vi "_set_mixer_params.vi"(9 "_LO_P_OPT":T2={"範囲配列"=[{"Start"=1.0, "Stop"=3.5, "Step"=0.1, "ｂｙ"="NEL VG"}, {"Start"=30.0, "Stop"=75.0, "Step"=1.0, "ｂｙ"="Motor"}, {"Start"=0.5, "Stop"=2.5, "Step"=0.1, "ｂｙ"="WCA VD"}], "Optimize"=0, "file_name"="LP_914.0_Tmin_100519.csv", "Save?"=FALSE, "measure"=2, "current(uA)"=40.0, "wait(ms)"=0, "IFfrq(GHz)"=8.0, "aveg"=10, "SISparam option"=2} {"SISparam option" items=["Volt and Current", "Volt only"]; "measure" items=["Pmax (only HOT)", "Tmin (HOT/COLD)", "C current"]; "Optimize" items=["Sweep", "黄金分割"]; "範囲配列"."Step" format="%.2f"; "範囲配列"."Stop" format="%.2f"; "範囲配列"."Start" format="%.2f"}, 10 "Control":T4={"GPIB_ATT"="28", "6501Dev#"=1, "GPIB_SP"="18", "GPIB_PM"="13", "GPIB_DSA"="11", "GPIB_DMM (TPD)"="23", "GPIB_MPI"="COM12", "mortor設定"=[{"Axis"=0, "ID"=0, "HIspeed"=200.0, "LOspeed"=100.0, "ACCEL(ms)"=100.0, "Sratio"=50.0, "フリーラン\n"=FALSE, "文字列"="DSB HOT/COLD"}, {"Axis"=1, "ID"=0, "HIspeed"=4.0, "LOspeed"=4.0, "ACCEL(ms)"=100.0, "Sratio"=50.0, "フリーラン\n"=TRUE, "文字列"="SubMM Att"}, {"Axis"=0, "ID"=0, "HIspeed"=200.0, "LOspeed"=100.0, "ACCEL(ms)"=100.0, "Sratio"=50.0, "フリーラン\n"=FALSE, "文字列"="MPI Port1"}, {"Axis"=1, "ID"=0, "HIspeed"=200.0, "LOspeed"=100.0, "ACCEL(ms)"=100.0, "Sratio"=50.0, "フリーラン\n"=FALSE, "文字列"="MPI Port2"}, {"Axis"=1, "ID"=0, "HIspeed"=200.0, "LOspeed"=100.0, "ACCEL(ms)"=100.0, "Sratio"=50.0, "フリーラン\n"=TRUE, "文字列"="gainComp"}], "DATAパス"=path "C:/Documents and Settings/band10/デスクトップ/data/cartridge/SN07/CCA07-11/120710_DSB", "mixer param file  "=path "C:/Documents and Settings/band10/デスクトップ/data/cartridge/SN07/120710_CCA07-11_mikxparam.csv", "comment"="120710_CCA07-11_DSB", "ColdCarts"="B10-07.11", "Th"=300.0, "Tc"=83.94, "Set_SIS_volt"=1.9, "Offset"=0.0, "control"=0, "FreqLO"=826.0, "Set_Mag_Cur"=9.66058394160584, "MPI offset(mm)"=23.128, "HOT/COLD"=0} {"HOT/COLD" items=["DSB", "SBR (Cart.)", "GainComp", "SBR (MIX)"]; "control" items=["CLOSE LOOP", "OPEN LOOP", "Not Control"]}, 11 "Bias_LO_equip":T3={"Node address"=19, "CAN Interface"="CAN0", "Cartridge band"=10, "Slave Node in"={"Address"=19, "Serial Number"=[16, 98, 22, 85, 1, 8, 0, 50]}, "ObjHandle out"=21, "POL"=1, "sb"=1, "GPIB_SM (SIS S,V)"="24", "GPIB_DMM (SIS I)"="22", "GPIB_SM (MAG I) "="25", "GPIB_SG(LO)"="19", "GPIB_PW (PAMP) "="6", "GPIB_TMP1(8ch)"="12", "GPIB_TMP2(2ch)  "="13", "WCA_avg"=10, "Rsen"=10.0, "BiasModule"=1, "LOModule "=2, "WCA_LO_FREQ_SET"={"YTO Low freq. [GHz]"=14.65, "YTO High freq. [GHz]"=17.5, "Kvco"=1, "Lock Pol."=0, "SET LO FREQ"=91.77778, "Multiplier"=6.0, "YTO (HEX)"=934, "YTO ( FREQ)"=15.300036, "NULL PLL INTEGRATOR"=FALSE}, "Res for"=0} {"Res for" items=["none", "series res", "parallel res"]; "WCA_LO_FREQ_SET"."YTO ( FREQ)" min=25 max=150 step=0.0001 format="%.3f"; "WCA_LO_FREQ_SET"."Multiplier" min=3 max=6 step=3; "WCA_LO_FREQ_SET"."SET LO FREQ" min=25 max=150 step=0.0001 format="%.3f"; "WCA_LO_FREQ_SET"."Lock Pol." items=["Lower", "Upper"]; "WCA_LO_FREQ_SET"."Kvco" items=["7.5MHz/V", "15MHz/V"]; "WCA_LO_FREQ_SET"."YTO High freq. [GHz]" format="%.3f"; "WCA_LO_FREQ_SET"."YTO Low freq. [GHz]" format="%.3f"; "LOModule" items=["Manual Gunn+PAMP"=0, "PLL GUNN+PAMP"=5, "B10Lab LO"=1, "WCA LO"=2, ""=3, "YIG発信器"=4, "none"=99]; "BiasModule" items=["B10Lab Bias"=0, "WCA BiasModule"=1, "none"=99]; "Slave Node in"."Serial Number" format="%.0x"; "Slave Node in"."Address" format="%.0x"; "Cartridge band" max=10 step=1; "Node address" format="%.0x"}) -> (1 "文字列":string="LOPt,826.00,1.31,1.84,21.22,-18.26,-21.13,146.13,19.78,,WCA,1.825867,205.642700,-0.241241,  3.501740,349.212646,-0.243988,", 2 "Control 2":T1={"GPIB_ATT"="28", "6501Dev#"=1, "GPIB_SP"="18", "GPIB_PM"="13", "GPIB_DSA"="11", "GPIB_DMM (TPD)"="23", "GPIB_MPI"="COM12", "mortor設定"=[{"Axis"=0, "ID"=0, "HIspeed"=200.0, "LOspeed"=100.0, "ACCEL(ms)"=100.0, "Sratio"=50.0, "フリーラン\n"=FALSE, "文字列"="DSB HOT/COLD"}, {"Axis"=1, "ID"=0, "HIspeed"=4.0, "LOspeed"=4.0, "ACCEL(ms)"=100.0, "Sratio"=50.0, "フリーラン\n"=TRUE, "文字列"="SubMM Att"}, {"Axis"=0, "ID"=0, "HIspeed"=200.0, "LOspeed"=100.0, "ACCEL(ms)"=100.0, "Sratio"=50.0, "フリーラン\n"=FALSE, "文字列"="MPI Port1"}, {"Axis"=1, "ID"=0, "HIspeed"=200.0, "LOspeed"=100.0, "ACCEL(ms)"=100.0, "Sratio"=50.0, "フリーラン\n"=FALSE, "文字列"="MPI Port2"}, {"Axis"=1, "ID"=0, "HIspeed"=200.0, "LOspeed"=100.0, "ACCEL(ms)"=100.0, "Sratio"=50.0, "フリーラン\n"=TRUE, "文字列"="gainComp"}], "DATAパス"=path "C:/Documents and Settings/band10/デスクトップ/data/cartridge/SN07/CCA07-11/120710_DSB", "DBパス "=path "C:/Documents and Settings/band10/デスクトップ/data/cartridge/SN07/120710_CCA07-11_mikxparam.csv", "comment"="120710_CCA07-11_DSB", "ColdCarts"="B10-07.11", "Th"=300.0, "Tc"=83.94, "Set_SIS_volt"=1.9, "Offset"=0.0, "control"=0, "FreqLO"=826.0, "Set_Mag_Cur"=9.66058394160584, "MPI offset(mm)"=23.128, "HOT/COLD"=0} {"HOT/COLD" items=["DSB", "SBR (Cart.)", "GainComp", "SBR (MIX)"]; "control" items=["CLOSE LOOP", "OPEN LOOP", "Not Control"]}, 3 "Bias_LO_equip 2":T3={"Node address"=19, "CAN Interface"="CAN0", "Cartridge band"=10, "Slave Node in"={"Address"=19, "Serial Number"=[16, 98, 22, 85, 1, 8, 0, 50]}, "ObjHandle out"=21, "POL"=1, "sb"=1, "GPIB_SM (SIS S,V)"="24", "GPIB_DMM (SIS I)"="22", "GPIB_SM (MAG I) "="25", "GPIB_SG(LO)"="19", "GPIB_PW (PAMP) "="6", "GPIB_TMP1(8ch)"="12", "GPIB_TMP2(2ch)  "="13", "WCA_avg"=10, "Rsen"=10.0, "BiasModule"=1, "LOModule "=2, "WCA_LO_FREQ_SET"={"YTO Low freq. [GHz]"=14.65, "YTO High freq. [GHz]"=17.5, "Kvco"=1, "Lock Pol."=0, "SET LO FREQ"=91.77778, "Multiplier"=6.0, "YTO (HEX)"=934, "YTO ( FREQ)"=15.300036, "NULL PLL INTEGRATOR"=FALSE}, "Res for"=0} {"Res for" items=["none", "series res", "parallel res"]; "WCA_LO_FREQ_SET"."YTO ( FREQ)" min=25 max=150 step=0.0001 format="%.4f"; "WCA_LO_FREQ_SET"."Multiplier" min=3 max=6 step=3; "WCA_LO_FREQ_SET"."SET LO FREQ" min=25 max=150 step=0.0001 format="%.3f"; "WCA_LO_FREQ_SET"."Lock Pol." items=["Lower", "Upper"]; "WCA_LO_FREQ_SET"."Kvco" items=["7.5MHz/V", "15MHz/V"]; "WCA_LO_FREQ_SET"."YTO High freq. [GHz]" format="%.3f"; "WCA_LO_FREQ_SET"."YTO Low freq. [GHz]" format="%.3f"; "LOModule" items=["Manual", "B10Lab LO", "WCA LO"]; "BiasModule" items=["B10Lab Bias", "WCA BiasModule"]; "Slave Node in"."Serial Number" format="%.0x"; "Slave Node in"."Address" format="%.0x"; "Cartridge band" max=10 step=1; "Node address" format="%.0x"})   [LabVIEW 2017]
uses:
  WCA_NAOJ_sub_vi/WCA_Global.vi
  <vilib>/Utility/file.llb/Read From Spreadsheet File (string).vi
  <vilib>/gmath/NI_Gmath.lvlib
panel:
  out "配列":string[][](array[string])=[["MixerParam", "4.46", "794", " 2012-07-10  09:04:23", "1.79", "41", "9.9", "", "", "1", "2", "1", "1.85", "0", "10.2", "0.32"], ["MixerParam", "4.46", "799", " 2012-07-10  09:09:38", "1.79", "41", "9.9", "", "", "1", "2", "1", "1.85", "0", "10.2", "0.32"], ["MixerParam", "4.46", "802", " 2012-07-10  09:14:53", "1.79", "41", "9.9", "", "", "1", "2", "1", "1.85", "0", "10.2", "0.32"], ["MixerParam", "4.46", "810", " 2012-07-10  09:20:08", "1.84", "41", "9.9", "", "", "1", "2", "1", "1.9", "0", "10.2", "0.32"], ["MixerParam", "4.46", "818", " 2012-07-10  09:25:23", "1.84", "41", "9.9", "", "", "1", "2", "1", "1.9", "0", "10.2", "0.32"], ["MixerParam", "4.46", "826", " 2012-07-10  09:30:38", "1.84", "41", "9.9", "", "", "1", "2", "1", "1.9", "0", "10.2", "0.33"], ["MixerParam", "4.46", "834", " 2012-07-10  09:35:53", "1.89", "41", "9.9", "", "", "1", "2", "1", "1.95", "0", "10.2", "0.32"], ["MixerParam", "4.46", "842", " 2012-07-10  09:41:08", "1.89", "41", "9.9", "", "", "1", "2", "1", "1.95", "0", "10.2", "0.33"], ["MixerParam", "4.47", "850", " 2012-07-10  09:46:24", "1.89", "41", "9.9", "", "", "1", "2", "1", "1.95", "0", "10.2", "0.32"], ["MixerParam", "4.46", "858", " 2012-07-10  09:51:42", "1.89", "41", "9.9", "", "", "1", "2", "1", "1.95", "0", "10.2", "0.32"], ["MixerParam", "4.46", "866", " 2012-07-10  09:56:58", "1.94", "41", "9.9", "", "", "1", "2", "1", "2", "0", "10.2", "0.32"], ["MixerParam", "4.46", "874", " 2012-07-10  10:02:15", "1.94", "41", "9.9", "", "", "1", "2", "1", "2", "0", "10.2", "0.32"], ["MixerParam", "4.46", "882", " 2012-07-10  10:07:32", "1.94", "41", "9.9", "", "", "1", "2", "1", "2", "0", "10.2", "0.32"], ["MixerParam", "4.47", "890", " 2012-07-10  10:12:49", "1.94", "41", "9.9", "", "", "1", "2", "1", "2", "0", "10.2", "0.32"], ["MixerParam", "4.46", "893", " 2012-07-10  10:18:06", "1.98", "41", "9.9", "", "", "1", "2", "1", "2.05", "0", "10.2", "0.32"], ["MixerParam", "4.46", "898", " 2012-07-10  10:23:23", "2", "41", "9.9", "", "", "1", "2", "1", "2.05", "0", "10.2", "0.32"], ["MixerParam", "4.46", "906", " 2012-07-10  10:28:43", "2", "41", "9.9", "", "", "1", "2", "1", "2.05", "0", "10.2", "0.32"], ["MixerParam", "4.46", "914", " 2012-07-10  10:34:01", "1.99", "41", "9.9", "", "", "1", "2", "1", "2.05", "0", "10.2", "0.33"], ["MixerParam", "4.46", "922", " 2012-07-10  10:39:20", "2.04", "41", "9.9", "", "", "1", "2", "1", "2.1", "0", "10.2", "0.32"], ["MixerParam", "4.46", "930", " 2012-07-10  10:44:38", "2.04", "41", "9.9", "", "", "1", "2", "1", "2.1", "0", "10.2", "0.32"], ["MixerParam", "4.46", "938", " 2012-07-10  10:49:56", "2.04", "41", "9.9", "", "", "1", "2", "1", "2.1", "0", "10.2", "0.32"]]
  out "set I":dbl=41.0
  out "set offset":dbl
  out "setV":dbl=1.9
  out "offset":dbl[](array[numeric])
  out "I":dbl[](array[numeric])=[41.0, 41.0, 41.0, 41.0, 41.0, 41.0, 41.0, 41.0, 41.0, 41.0, 41.0, 41.0, 41.0, 41.0, 41.0, 41.0, 41.0, 41.0, 41.0, 41.0, 41.0]
  out "V":dbl[](array[numeric])=[1.85, 1.85, 1.85, 1.9, 1.9, 1.9, 1.95, 1.95, 1.95, 1.95, 2.0, 2.0, 2.0, 2.0, 2.05, 2.05, 2.05, 2.05, 2.1, 2.1, 2.1]
  out "LO":dbl[](array[numeric])=[794.0, 799.0, 802.0, 810.0, 818.0, 826.0, 834.0, 842.0, 850.0, 858.0, 866.0, 874.0, 882.0, 890.0, 893.0, 898.0, 906.0, 914.0, 922.0, 930.0, 938.0]
  out "Link済み":bool=TRUE
  # "LO freq. [GHz]"
  # "YTO LOW\n/High Freq."
  # "ZERO Intgrtr"
  # "Node Address"
  # "Serial Number"
  # "LO freq. [GHz]"
  # "YTO LOW\n/High Freq."
  # "ZERO Intgrtr"
  # "Node Address"
  # "Serial Number"
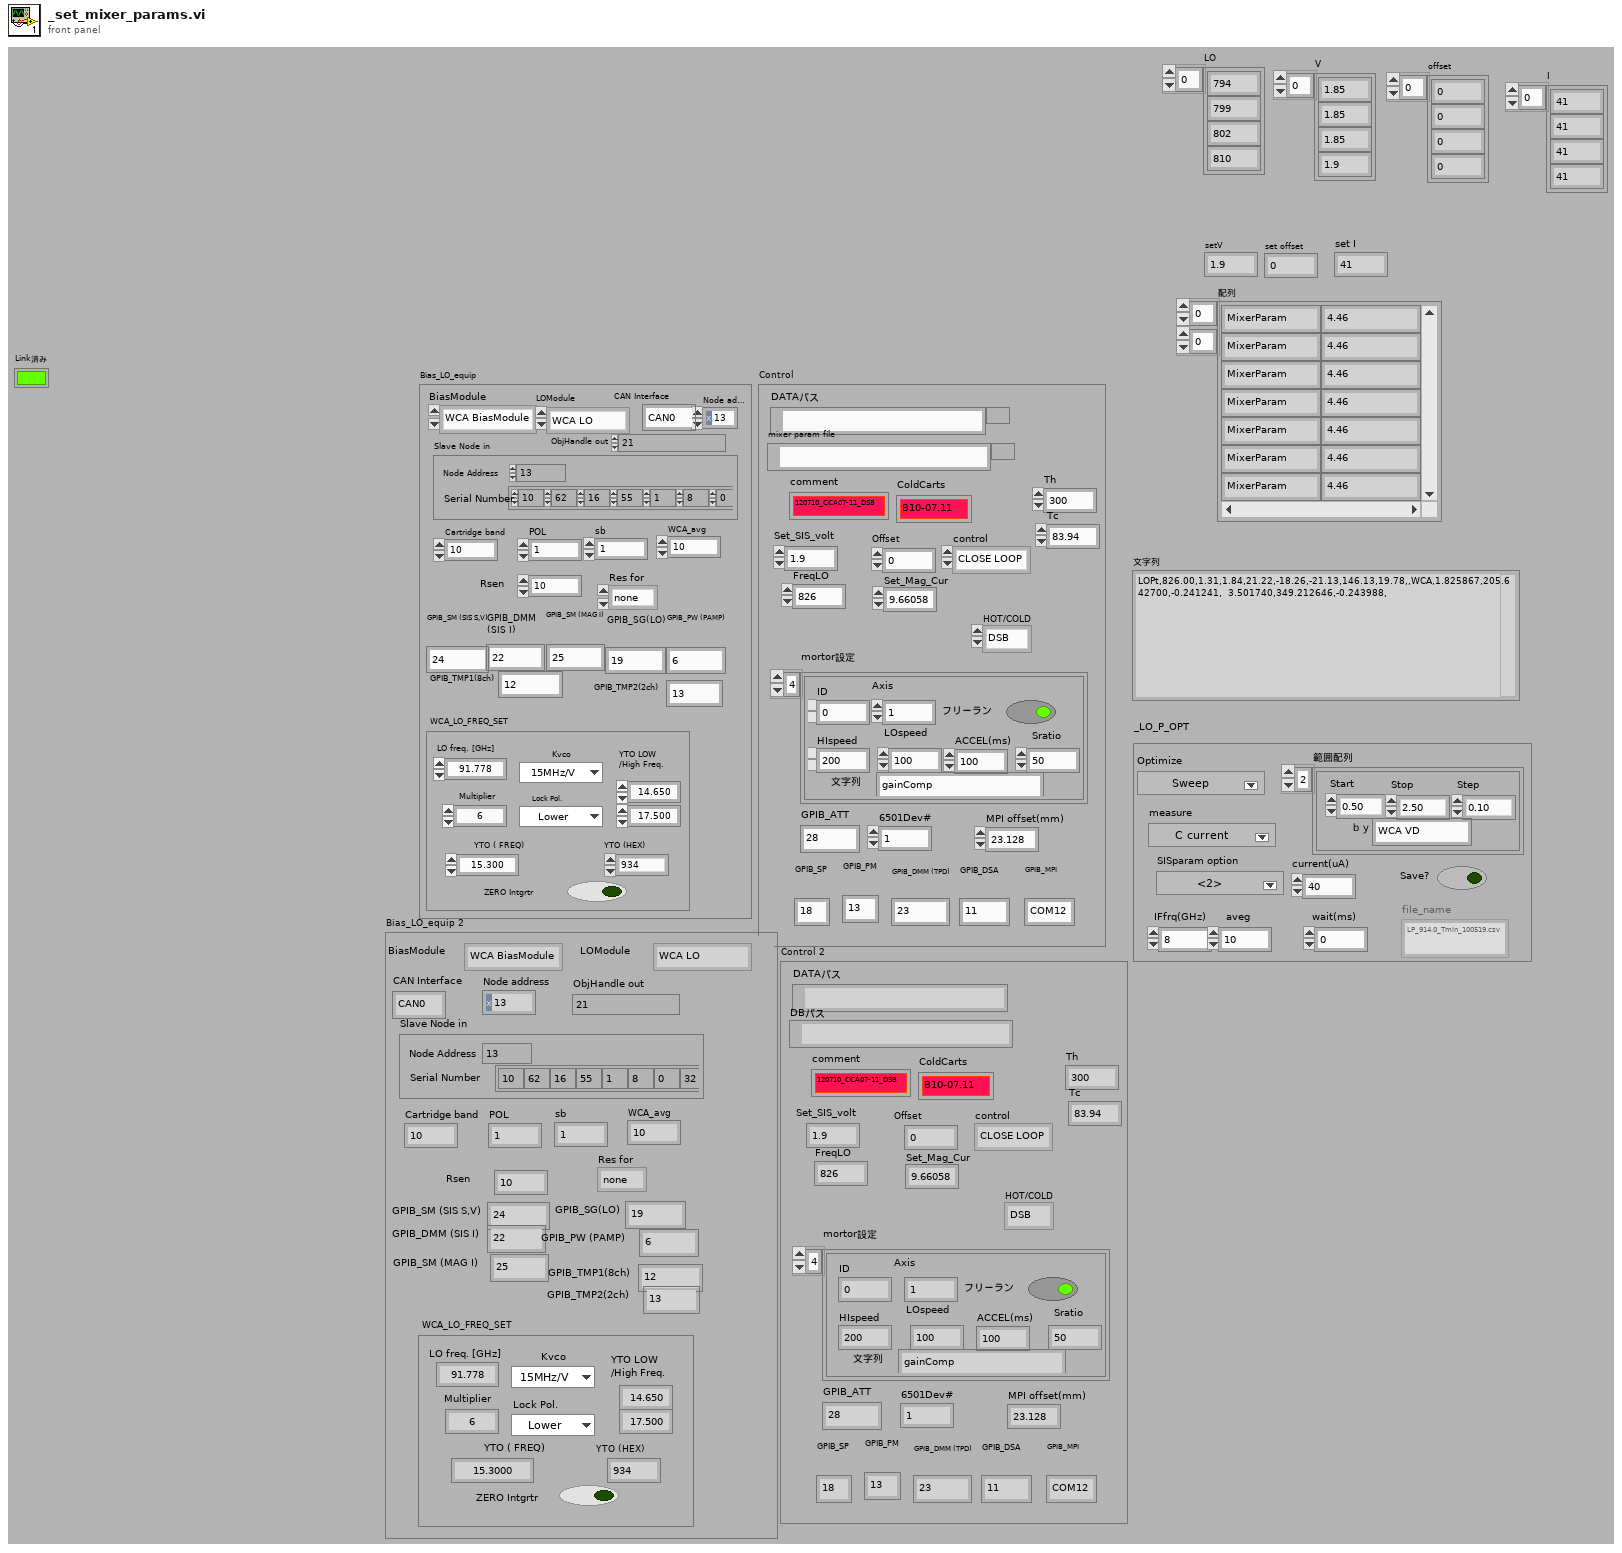
[diagram p1: front panel]
types:
  T1 = cluster{"GPIB_ATT":string, "6501Dev#":i16, "GPIB_SP":string, "GPIB_PM":string, "GPIB_DSA":string, "GPIB_DMM (TPD)":string, "GPIB_MPI":string, "mortor設定":cluster{"Axis":i16, "ID":i16, "HIspeed":dbl, "LOspeed":dbl, "ACCEL(ms)":dbl, "Sratio":dbl, "フリーラン\n":bool, "文字列":string}[], "DATAパス":path, "DBパス ":path, "comment":string, "ColdCarts":string, "Th":dbl, "Tc":dbl, "Set_SIS_volt":dbl, "Offset":dbl, "control":u16, "FreqLO":dbl, "Set_Mag_Cur":dbl, "MPI offset(mm)":dbl, "HOT/COLD":u16}
  T2 = cluster{"範囲配列":cluster{"Start":dbl, "Stop":dbl, "Step":dbl, "ｂｙ":string}[], "Optimize":u16, "file_name":string, "Save?":bool, "measure":u16, "current(uA)":dbl, "wait(ms)":i32, "IFfrq(GHz)":dbl, "aveg":i32, "SISparam option":u16}
  T3 = cluster{"Node address":u16, "CAN Interface":string, "Cartridge band":u32, "Slave Node in":cluster{"Address":i16, "Serial Number":i8[]}, "ObjHandle out":u32, "POL":u32, "sb":u32, "GPIB_SM (SIS S,V)":string, "GPIB_DMM (SIS I)":string, "GPIB_SM (MAG I) ":string, "GPIB_SG(LO)":string, "GPIB_PW (PAMP) ":string, "GPIB_TMP1(8ch)":string, "GPIB_TMP2(2ch)  ":string, "WCA_avg":i32, "Rsen":dbl, "BiasModule":u16, "LOModule ":u16, "WCA_LO_FREQ_SET":cluster{"YTO Low freq. [GHz]":sgl, "YTO High freq. [GHz]":sgl, "Kvco":u16, "Lock Pol.":u16, "SET LO FREQ":sgl, "Multiplier":sgl, "YTO (HEX)":u16, "YTO ( FREQ)":sgl, "NULL PLL INTEGRATOR":bool}, "Res for":u16}
  T4 = cluster{"GPIB_ATT":string, "6501Dev#":i16, "GPIB_SP":string, "GPIB_PM":string, "GPIB_DSA":string, "GPIB_DMM (TPD)":string, "GPIB_MPI":string, "mortor設定":cluster{"Axis":i16, "ID":i16, "HIspeed":dbl, "LOspeed":dbl, "ACCEL(ms)":dbl, "Sratio":dbl, "フリーラン\n":bool, "文字列":string}[], "DATAパス":path, "mixer param file  ":path, "comment":string, "ColdCarts":string, "Th":dbl, "Tc":dbl, "Set_SIS_volt":dbl, "Offset":dbl, "control":u16, "FreqLO":dbl, "Set_Mag_Cur":dbl, "MPI offset(mm)":dbl, "HOT/COLD":u16}
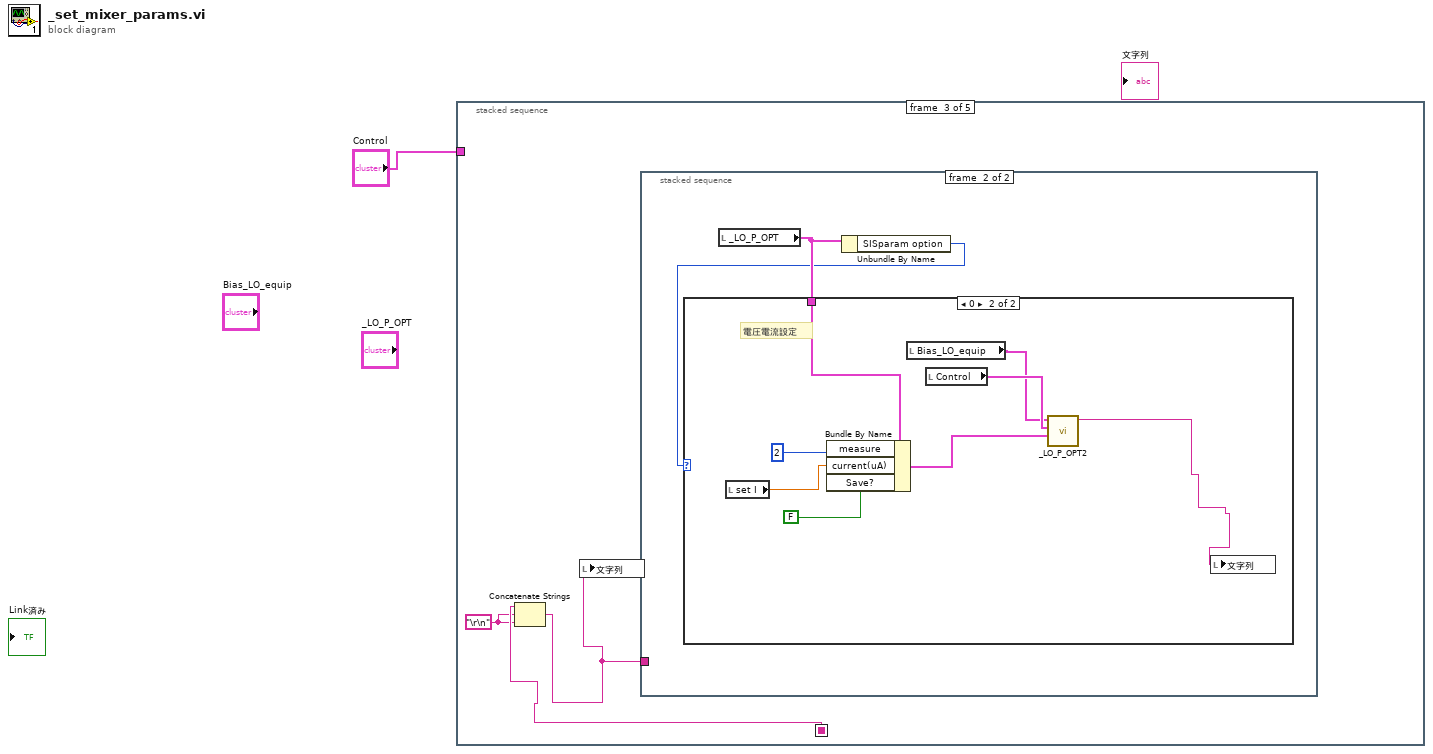
[diagram p0: block diagram]
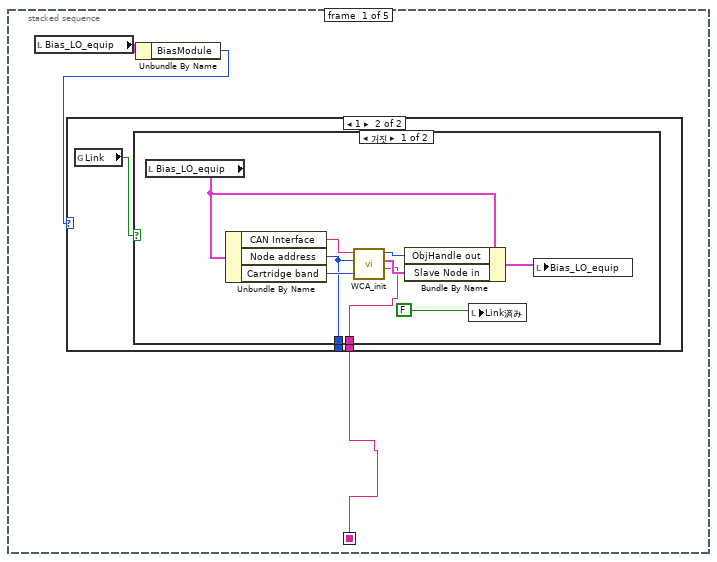
[diagram p2: hidden frame]
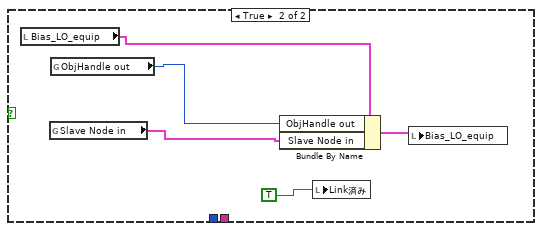
[diagram p4: hidden frame]
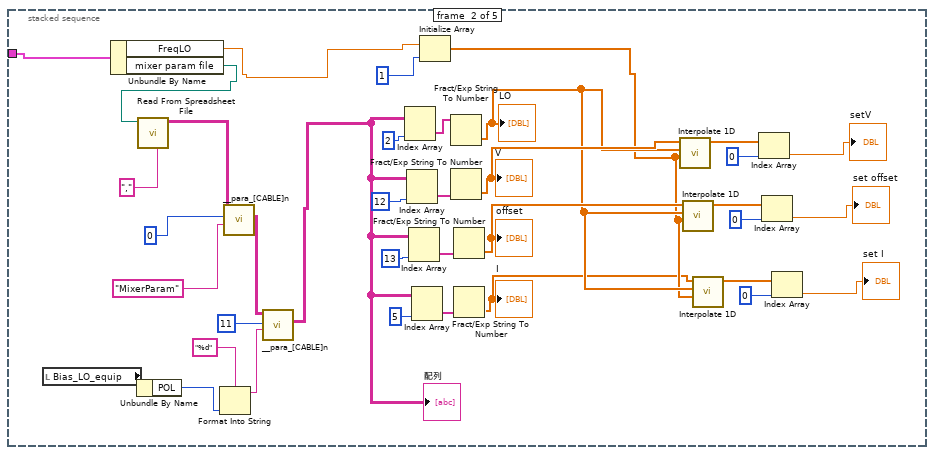
[diagram p5: hidden frame]
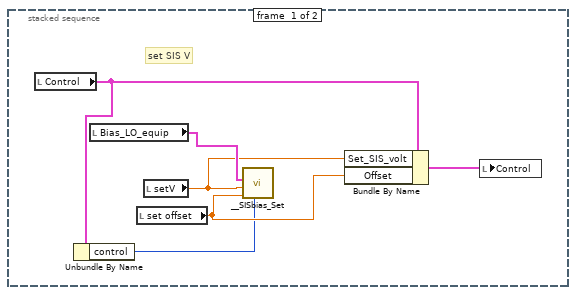
[diagram p6: hidden frame]
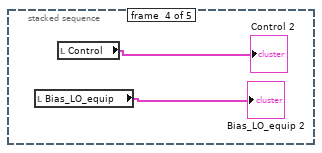
[diagram p8: hidden frame]
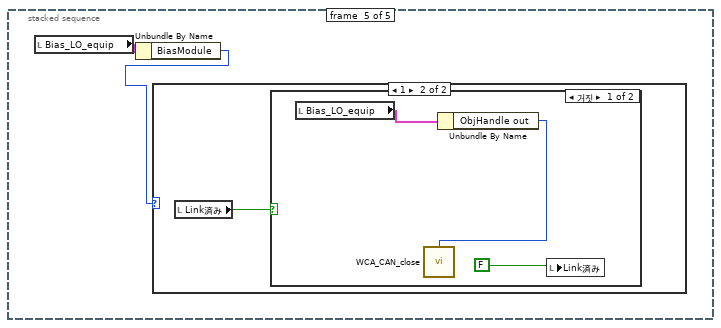
[diagram p9: hidden frame]
diagram:
  n1 = stacked-sequence {
    seq-local: [w2 _ _ _ _] -> [_ _ w61 _ _]
    tunnel: "Control" -> [_ w27 _ _ _]
    frame #0 {
      n2 = local read "Bias_LO_equip"() -> (w4:T3)
      n3 = Unbundle By Name(w4) -> ("BiasModule"=w3:u16)
      n4 = case shown="1" w3 {
        tunnel: [_ w6] -> w2
        tunnel: [_ w5] -> _
        frame 0, Default {
        }
        frame 1 {
          n5 = global read "WCA_Global.vi" "Link"() -> (w7:bool)
          n6 = case shown="거짓" w7 {
            tunnel: [w8 _] -> w6
            tunnel: [w9 _] -> w5
            frame False {
              n7 = local read "Bias_LO_equip"() -> (w10:T3)
              n8 = Unbundle By Name(w10) -> ("CAN Interface"=w13:string, "Node address"=w9:u16, "Cartridge band"=w12:u32)
              n9 = call "WCA_init.vi"("Cartridge band"=w12, "Node address"=w9, "CAN Interface"=w13) -> ("Detected CAN Nodes."=w8:string, "Slave Node in"=w15:cluster{"Address":i16, "Serial Number":i8[]}, "ObjHandle out"=w16:u32)  [unwired: 4 in, 2 out]
              n10 = Bundle By Name(cluster=w10, "ObjHandle out"=w16, "Slave Node in"=w15) -> (w11:T3)
              n11 = local write "Link済み"(FALSE) -> ()
              n12 = local write "Bias_LO_equip"(w11) -> ()
            }
            frame True {
              n13 = local read "Bias_LO_equip"() -> (w20:T3)
              n14 = global read "WCA_Global.vi" "Slave Node in"() -> (w18:cluster{"Address":i16, "Serial Number":i8[]})
              n15 = global read "WCA_Global.vi" "ObjHandle out"() -> (w19:u32)
              n16 = Bundle By Name(cluster=w20, "ObjHandle out"=w19, "Slave Node in"=w18) -> (w21:T3)
              n17 = local write "Link済み"(TRUE) -> ()
              n18 = local write "Bias_LO_equip"(w21) -> ()
            }
          }
        }
      }
    }
    frame #1 {
      n19 = local read "Bias_LO_equip"() -> (w32:T3)
      n20 = Unbundle By Name(w27) -> ("FreqLO"=w26:dbl, "mixer param file"=w22:path)
      n21 = Unbundle By Name(w32) -> ("POL"=w31:u32)
      n22 = call-poly <vilib>:"Read From Spreadsheet File.vi"("delimiter (\\t)"=",", "file path (dialog if empty)"=w22) -> ("all rows"=w37:string[][])  [unwired: 5 in, 4 out]
      n23 = Format Into String(format string="%d", w31) -> (resulting string=w29:string)  [unwired: 2 in, 1 out]
      n24 = call "__para_[CABLE]n.vi"("検索値"="MixerParam", "検索キー列"=0, "読み込み配列"=w37) -> ("出力配列"=w34:string[][])  [unwired: 6 in]
      n25 = call "__para_[CABLE]n.vi"("検索値"=w29, "検索キー列"=11, "読み込み配列"=w34) -> ("出力配列"=w33:string[][])  [unwired: 6 in]
      "配列" <- w33
      n26 = Index Array(array=w33, index (col)=2) -> (element=w56:string[])  [unwired: 1 in]
      n27 = Index Array(array=w33, index (col)=12) -> (element=w54:string[])  [unwired: 1 in]
      n28 = Index Array(array=w33, index (col)=13) -> (element=w50:string[])  [unwired: 1 in]
      n29 = Index Array(array=w33, index (col)=5) -> (element=w52:string[])  [unwired: 1 in]
      n30 = Initialize Array(w26, 1) -> (w39:dbl[])
      n31 = Fract/Exp String To Number(string=w56) -> (number=w40:dbl[])  [unwired: 3 in, 1 out]
      "LO" <- w40
      n32 = Fract/Exp String To Number(string=w54) -> (number=w49:dbl[])  [unwired: 3 in, 1 out]
      "V" <- w49
      n33 = Fract/Exp String To Number(string=w50) -> (number=w41:dbl[])  [unwired: 3 in, 1 out]
      "offset" <- w41
      n34 = Fract/Exp String To Number(string=w52) -> (number=w38:dbl[])  [unwired: 3 in, 1 out]
      "I" <- w38
      n35 = call <vilib>:"Interpolate 1D.vi"("xi"=w39, "X"=w40, "Y"=w49) -> ("yi"=w48:dbl[])  [unwired: 6 in, 2 out]
      n36 = call <vilib>:"Interpolate 1D.vi"("xi"=w39, "X"=w40, "Y"=w41) -> ("yi"=w45:dbl[])  [unwired: 6 in, 2 out]
      n37 = call <vilib>:"Interpolate 1D.vi"("xi"=w39, "X"=w40, "Y"=w38) -> ("yi"=w43:dbl[])  [unwired: 6 in, 2 out]
      n38 = Index Array(array=w48, index=0) -> (element=→"setV":dbl)
      n39 = Index Array(array=w45, index=0) -> (element=→"set offset":dbl)
      n40 = Index Array(array=w43, index=0) -> (element=→"set I":dbl)
    }
    frame #2 {
      w60 = "\r\n"
      n41 = Concatenate Strings(w61, w60, w60) -> (w59:string)
      n42 = local write "文字列"(w59) -> ()
      n43 = stacked-sequence {
        tunnel: w59 -> [_ _]
        frame #0 {
          # "set SIS V"
          n44 = local read "Control"() -> (w63:T4)
          n45 = Unbundle By Name(w63) -> ("control"=w62:u16)
          n46 = local read "Bias_LO_equip"() -> (w67:T3)
          n47 = local read "set offset"() -> (w64:dbl)
          n48 = local read "setV"() -> (w65:dbl)
          n49 = call "__SISbias_Set.vi"("SIS　Mode"=w62, "Offset"=w64, "Set_V"=w65, "Bias_LO_equip"=w67) -> ()  [unwired: 7 in, 1 out]
          n50 = Bundle By Name(cluster=w63, "Set_SIS_volt"=w65, "Offset"=w64) -> (w66:T4)
          n51 = local write "Control"(w66) -> ()
        }
        frame #1 {
          n52 = local read "_LO_P_OPT"() -> (w69:T2)
          n53 = Unbundle By Name(w69) -> ("SISparam option"=w68:u16)
          n54 = case shown="0" w68 {
            tunnel: w69 -> [_ w70]
            frame 1, Default {
              # "電圧のみ設定"
            }
            frame 0 {
              # "電圧電流設定"
              n55 = local read "set I"() -> (w76:dbl)
              n56 = Bundle By Name(cluster=w70, "measure"=2, "current(uA)"=w76, "Save?"=FALSE) -> (w74:T2)
              n57 = local read "Bias_LO_equip"() -> (w72:T3)
              n58 = local read "Control"() -> (w73:T4)
              n59 = call "_LO_P_OPT2.vi"("_LO_P_OPT"=w74, "Control"=w73, "Bias_LO_equip"=w72) -> ("結果"=w71:string)  [unwired: 4 in]
              n60 = local write "文字列"(w71) -> ()
            }
          }
        }
      }
    }
    frame #3 {
      n61 = local read "Bias_LO_equip"() -> (→"Bias_LO_equip 2":T3)
      n62 = local read "Control"() -> (→"Control 2":T4)
    }
    frame #4 {
      n63 = local read "Bias_LO_equip"() -> (w81:T3)
      n64 = Unbundle By Name(w81) -> ("BiasModule"=w80:u16)
      n65 = case shown="1" w80 {
        frame 0, Default {
        }
        frame 1 {
          n66 = local read "Link済み"() -> (w82:bool)
          n67 = case shown="거짓" w82 {
            frame False {
              n68 = local read "Bias_LO_equip"() -> (w84:T3)
              n69 = Unbundle By Name(w84) -> ("ObjHandle out"=w83:u32)
              n70 = call "WCA_CAN_close.vi"("ObjHandle in"=w83) -> ()  [unwired: 14 in, 1 out]
              n71 = local write "Link済み"(FALSE) -> ()
            }
            frame True {
            }
          }
        }
      }
    }
  }
